vi "Read Data.vi"(3 "Read Data":bool, 4 "Chosen com is opened!":bool, 5 "VISA resource name":refnum<visa-resource-name>) -> (0 "error while reading":bool, 1 "Data":u8[](array[numeric]) format="%x", 2 "VISA resource name out":refnum<visa-resource-name>)   [LabVIEW 2020]
panel:
  in  "byte count":u32=5
  out "element":u8
  out "unsigned byte array":u8[](array[numeric])
  out "return count":u32
  out "reader2":bool
  out "reader1":bool
  out "read data is enable?":bool
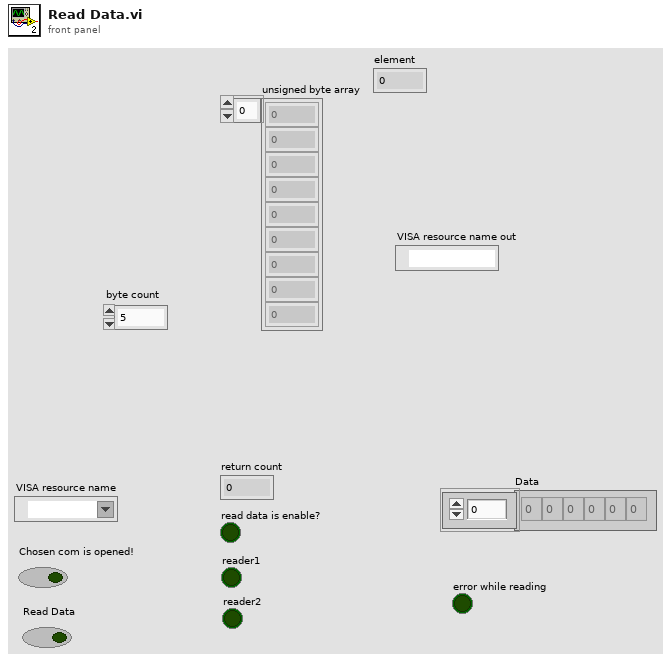
[diagram p1: front panel]
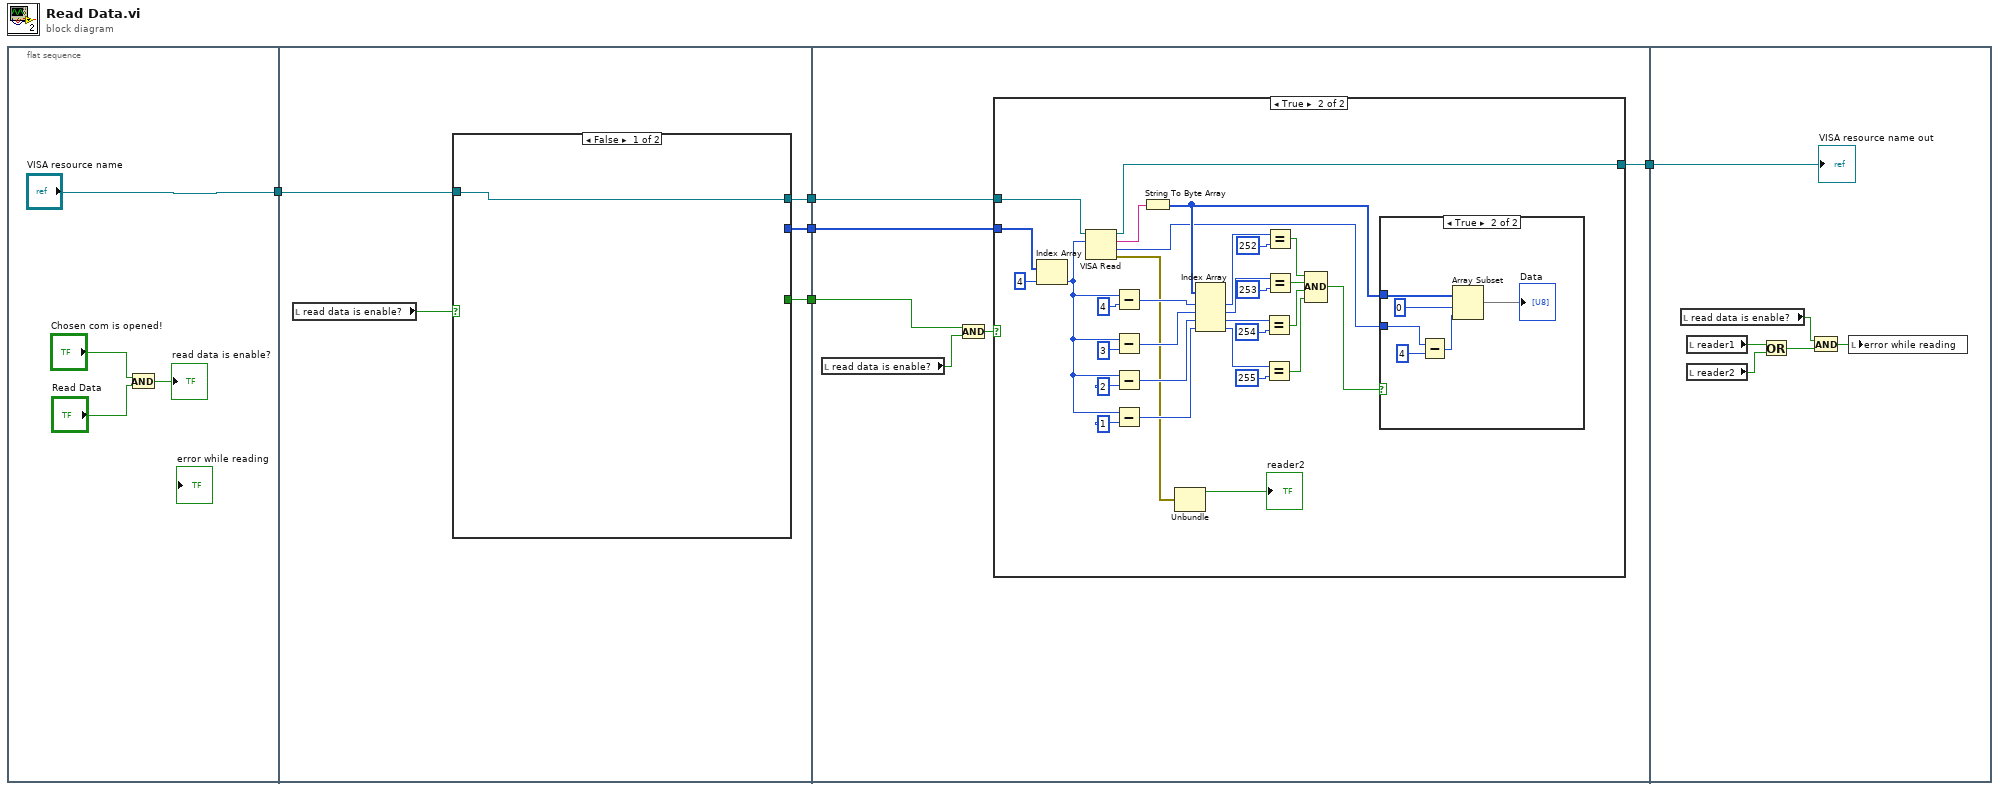
[diagram p0: block diagram]
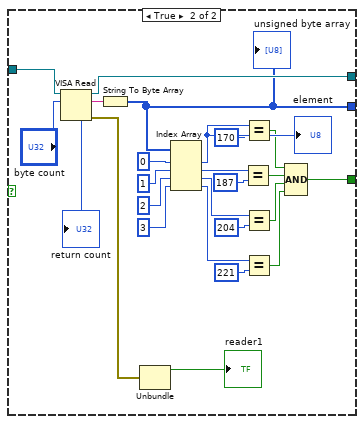
[diagram p2: hidden frame]
diagram:
  n1 = flat-sequence {
    tunnel: ["VISA resource name"] -> w4
    tunnel: [w14] -> w5
    tunnel: w4 -> [w13]
    tunnel: [w12] -> w3
    tunnel: [w10] -> w2
    tunnel: w5 -> [w46]
    tunnel: w3 -> [w45]
    tunnel: w2 -> [w43]
    tunnel: [w41] -> w1
    tunnel: w1 -> [w85]
    frame #0 {
      n2 = And(x="Chosen com is opened!", y="Read Data") -> (x .and. y?=→"read data is enable?":bool)
    }
    frame #1 {
      n3 = local read "read data is enable?"() -> (w11:bool)
      n4 = case shown="False" w11 {
        tunnel: [w15 w39] -> w14
        tunnel: w13 -> [w15 w21]
        tunnel: [_ w20] -> w12
        tunnel: [_ w19] -> w10
        frame False {
        }
        frame True {
          n5 = VISA Read(VISA resource name=w21, byte count="byte count") -> (VISA resource name out=w39:refnum<visa-resource-name>, read buffer=w22:string, return count=→"return count":u32, error out=w18:errorcluster)  [unwired: 1 in]
          n6 = String To Byte Array(string=w22) -> (unsigned byte array=w20:u8[])
          "unsigned byte array" <- w20
          n7 = Unbundle(w18) -> ("status"=→"reader1":bool)  [unwired: 2 out]
          n8 = Index Array(array=w20, index #1=0 ("index"), index #2=1 ("index"), index #3=2 ("index"), index #4=3 ("index")) -> (element #1=w34:u8, element #2=w33:u8, element #3=w32:u8, element #4=w31:u8)
          "element" <- w34
          n9 = Equal?(x=w33, y=u8 187 ("H3")) -> (x = y?=w29:bool)
          n10 = Equal?(x=w34, y=u8 170 ("H1")) -> (x = y?=w30:bool)
          n11 = Equal?(x=w32, y=u8 204 ("H2")) -> (x = y?=w28:bool)
          n12 = Equal?(x=w31, y=u8 221 ("H4")) -> (x = y?=w27:bool)
          n13 = Compound Arithmetic op=AND(w30, w29, w28, w27) -> (w19:bool)
        }
      }
    }
    frame #2 {
      n14 = local read "read data is enable?"() -> (w44:bool)
      n15 = And(x=w43, y=w44) -> (x .and. y?=w42:bool)
      n16 = case shown="True" w42 {
        tunnel: w46 -> [w47 w52]
        tunnel: w45 -> [_ w51]
        tunnel: [w47 w48] -> w41
        frame False {
        }
        frame True {
          n17 = Index Array(array=w51, index=4) -> (element=w54:u8)
          n18 = VISA Read(VISA resource name=w52, byte count=w54) -> (VISA resource name out=w48:refnum<visa-resource-name>, read buffer=w78:string, return count=w53:u32, error out=w50:errorcluster)  [unwired: 1 in]
          n19 = Subtract(x=w54, y=u8 4) -> (x-y=w76:u8)
          n20 = Subtract(x=w54, y=u8 3) -> (x-y=w75:u8)
          n21 = Subtract(x=w54, y=u8 2) -> (x-y=w74:u8)
          n22 = Subtract(x=w54, y=u8 1) -> (x-y=w73:u8)
          n23 = String To Byte Array(string=w78) -> (unsigned byte array=w59:u8[])
          n24 = Unbundle(w50) -> ("status"=→"reader2":bool)  [unwired: 2 out]
          n25 = Index Array(array=w59, index #1=w76, index #2=w75, index #3=w74, index #4=w73) -> (element #1=w68:u8, element #2=w67:u8, element #3=w66:u8, element #4=w65:u8)
          n26 = Equal?(x=w66, y=u8 254 ("F3")) -> (x = y?=w62:bool)
          n27 = Equal?(x=w65, y=u8 255 ("F4")) -> (x = y?=w61:bool)
          n28 = Equal?(x=w68, y=u8 252 ("F1")) -> (x = y?=w64:bool)
          n29 = Equal?(x=w67, y=u8 253 ("F2")) -> (x = y?=w63:bool)
          n30 = Compound Arithmetic op=AND(w64, w63, w62, w61) -> (w60:bool)
          n31 = case shown="True" w60 {
            tunnel: w53 -> [_ w81]
            tunnel: w59 -> [_ w83]
            frame False {
            }
            frame True {
              n32 = Subtract(x=w81, y=u8 4) -> (x-y=w79:u32)
              n33 = Array Subset(array=w83, index=0, length=w79) -> (→"Data":u8[])
            }
          }
        }
      }
    }
    frame #3 {
      n34 = local read "read data is enable?"() -> (w88:bool)
      n35 = local read "reader1"() -> (w90:bool)
      n36 = local read "reader2"() -> (w89:bool)
      n37 = Or(x=w90, y=w89) -> (x .or. y?=w87:bool)
      n38 = And(x=w88, y=w87) -> (x .and. y?=w86:bool)
      n39 = local write "error while reading"(w86) -> ()
      "VISA resource name out" <- w85
    }
  }
